vi "libssh2_exit.vi"(8 "error in (no error)":errorcluster) -> (0 "error out":errorcluster)   [LabVIEW 2013, in "libssh2.lvlib"]
uses:
  libssh2.lvlib
  libssh2.dll
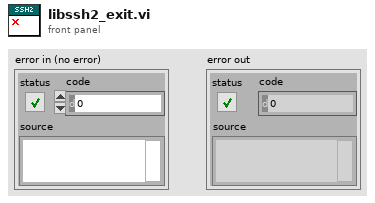
[diagram p1: front panel]
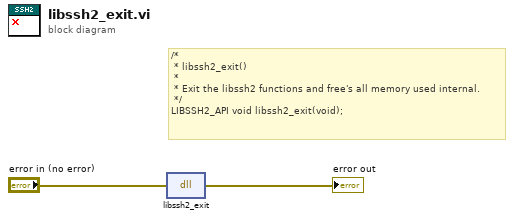
[diagram p0: block diagram]
diagram:
  # "/*\n * libssh2_exit()\n *\n * Exit the libssh2 functions and free's all memory used internal.\n */\nLIBSSH2_API void libssh2_exit(void);"
  n1 = dll-call lib="C:/Users/pasca/OneDrive/LabVIEW/libssh2/libssh2**.*" fn="libssh2_exit"(error in="error in (no error)") -> (error out=→"error out":errorcluster)  [unwired: 3 in, 1 out]
